vi "oscilloscope.vi"() -> ()   [LabVIEW 2023]
uses:
  <vilib>/LabVIEW Targets/FPGA/cRIO/shared/nicrio_ModuleControls/nicrio_BasicConversionTime.ctl
  <vilib>/LabVIEW Targets/FPGA/cRIO/shared/nicrio_ModuleControls/nicrio_cRIO-9775_RecordDataRates4ChansRing.ctl
  <vilib>/rvi/Emulation/niFpgaGetClockAttributes.vi
  <vilib>/rvi/Emulation/niFpgaSctlEmulationGetInTimedLoop.vi
  <vilib>/rvi/Emulation/niFpgaEmulationReportErrorSimple.vi
  <vilib>/rvi/Emulation/niFpgaProcessEmulError.vi
  <vilib>/rvi/eio/common/nirviEmuTemplateMethod_errors.vi
  <vilib>/rvi/Emulation/niFpgaCriticalErrorInLSC.vi
  <vilib>/rvi/eio/common/nirviEmuTemplatePropertySet_errors.vi
  <vilib>/eio/EIONode/EIONode.xnode
  <vilib>/eio/EIOPropertyNode/EIOPropertyNode.xnode
  <vilib>/eio/EIOMethodNode/EIOMethodNode.xnode
  <vilib>/rvi/eio/common/nirviEmuTemplatePropertyGet_errors.vi
  <vilib>/rvi/eio/common/nirviEmuTemplatePropertyGet_noerrors.vi
  <vilib>/rvi/eio/common/nirviEmuTemplatePropertySet_noerrors.vi
panel:
  in  "Reading channel":T1={"Chan 0"=TRUE, "Chan 1"=TRUE, "Chan 2"=TRUE, "Chan 3"=TRUE}
  in  "Record Samples":u32=1000000
  in  "Record Data Rate":T2=1 items=["20.000 MS/s (NI 9775)"=1, "10.00 MS/s (NI 9775)"=2, "6.667 MS/s (NI 9775)"=3, "5.000 MS/s (NI 9775)"=4, "2.500 MS/s (NI 9775)"=8, "1.667 MS/s (NI 9775)"=12, "1.250 MS/s (NI 9775)"=16, "1.000 MS/s (NI 9775)"=20, "833.333 KS/s (NI 9775)"=24, "714.286 KS/s (NI 9775)"=28, "625.000 KS/s (NI 9775)"=32, "555.556 KS/s (NI 9775)"=36, "500.000 KS/s (NI 9775)"=40, "454.545 KS/s (NI 9775)"=44, "416.667 KS/s (NI 9775)"=48, "384.615 KS/s (NI 9775)"=52, "357.143 KS/s (NI 9775)"=56, "333.333 KS/s (NI 9775)"=60, "312.500 KS/s (NI 9775)"=64, "294.118 KS/s (NI 9775)"=68, "277.778 KS/s (NI 9775)"=72, "263.158 KS/s (NI 9775)"=76, "250.000 KS/s (NI 9775)"=80, "238.095 KS/s (NI 9775)"=84, "227.273 KS/s (NI 9775)"=88, "217.391 KS/s (NI 9775)"=92, "208.333 KS/s (NI 9775)"=96, "200.000 KS/s (NI 9775)"=100, "192.308 KS/s (NI 9775)"=104, "185.185 KS/s (NI 9775)"=108, "178.571 KS/s (NI 9775)"=112, "172.414 KS/s (NI 9775)"=116, "166.667 KS/s (NI 9775)"=120, "161.290 KS/s (NI 9775)"=124, "156.250 KS/s (NI 9775)"=128, "151.515 KS/s (NI 9775)"=132, "147.059 KS/s (NI 9775)"=136, "142.857 KS/s (NI 9775)"=140, "138.889 KS/s (NI 9775)"=144, "135.135 KS/s (NI 9775)"=148, "131.579 KS/s (NI 9775)"=152, "128.205 KS/s (NI 9775)"=156, "125.000 KS/s (NI 9775)"=160, "121.951 KS/s (NI 9775)"=164, "119.048 KS/s (NI 9775)"=168, "116.279 KS/s (NI 9775)"=172, "113.636 KS/s (NI 9775)"=176, "111.111 KS/s (NI 9775)"=180, "108.696 KS/s (NI 9775)"=184, "106.383 KS/s (NI 9775)"=188, "104.167 KS/s (NI 9775)"=192, "102.041 KS/s (NI 9775)"=196, "100.000 KS/s (NI 9775)"=200, "50.000 KS/s (NI 9775)"=400, "33.333 KS/s (NI 9775)"=600, "25.000 KS/s (NI 9775)"=800, "20.000 KS/s (NI 9775)"=1000, "16.667 KS/s (NI 9775)"=1200, "14.286 KS/s (NI 9775)"=1400, "12.500 KS/s (NI 9775)"=1600, "11.111 KS/s (NI 9775)"=1800, "10.000 KS/s (NI 9775)"=2000, "9.091 KS/s (NI 9775)"=2200, "8.333 KS/s (NI 9775)"=2400, "7.692 KS/s (NI 9775)"=2600, "7.143 KS/s (NI 9775)"=2800, "6.667 KS/s (NI 9775)"=3000, "6.250 KS/s (NI 9775)"=3200, "5.882 KS/s (NI 9775)"=3400, "5.556 KS/s (NI 9775)"=3600, "5.000 KS/s (NI 9775)"=4000, "4.762 KS/s (NI 9775)"=4200, "4.545 KS/s (NI 9775)"=4400, "4.348 KS/s (NI 9775)"=4600, "4.167 KS/s (NI 9775)"=4800, "4.000 KS/s (NI 9775)"=5000, "3.846 KS/s (NI 9775)"=5200, "3.571 KS/s (NI 9775)"=5600, "3.333 KS/s (NI 9775)"=6000, "3.125 KS/s (NI 9775)"=6400, "2.941 KS/s (NI 9775)"=6800, "2.778 KS/s (NI 9775)"=7200, "2.632 KS/s (NI 9775)"=7600, "2.500 KS/s (NI 9775)"=8000, "2.381 KS/s (NI 9775)"=8400, "2.273 KS/s (NI 9775)"=8800, "2.174 KS/s (NI 9775)"=9200, "2.083 KS/s (NI 9775)"=9600, "2.000 KS/s (NI 9775)"=10000, "1.923 KS/s (NI 9775)"=10400, "1.852 KS/s (NI 9775)"=10800, "1.786 KS/s (NI 9775)"=11200, "1.724 KS/s (NI 9775)"=11600, "1.667 KS/s (NI 9775)"=12000, "1.613 KS/s (NI 9775)"=12400, "1.563 KS/s (NI 9775)"=12800, "1.515 KS/s (NI 9775)"=13200, "1.471 KS/s (NI 9775)"=13600, "1.429 KS/s (NI 9775)"=14000, "1.389 KS/s (NI 9775)"=14400, "1.351 KS/s (NI 9775)"=14800, "1.316 KS/s (NI 9775)"=15200, "1.282 KS/s (NI 9775)"=15600, "1.250 KS/s (NI 9775)"=16000, "1.220 KS/s (NI 9775)"=16400, "1.190 KS/s (NI 9775)"=16800, "1.163 KS/s (NI 9775)"=17200, "1.136 KS/s (NI 9775)"=17600, "1.111 KS/s (NI 9775)"=18000, "1.087 KS/s (NI 9775)"=18400, "1.064 KS/s (NI 9775)"=18800, "1.042 KS/s (NI 9775)"=19200, "1.020 KS/s (NI 9775)"=19600, "1.000 KS/s (NI 9775)"=20000, "0.980 KS/s (NI 9775)"=20400, "0.962 KS/s (NI 9775)"=20800, "0.943 KS/s (NI 9775)"=21200, "0.926 KS/s (NI 9775)"=21600, "0.909 KS/s (NI 9775)"=22000, "0.893 KS/s (NI 9775)"=22400, "0.877 KS/s (NI 9775)"=22800, "0.862 KS/s (NI 9775)"=23200, "0.847 KS/s (NI 9775)"=23600, "0.833 KS/s (NI 9775)"=24000, "0.820 KS/s (NI 9775)"=24400, "0.806 KS/s (NI 9775)"=24800, "0.794 KS/s (NI 9775)"=25200, "0.781 KS/s (NI 9775)"=25600, "0.694 KS/s (NI 9775)"=28800, "0.625 KS/s (NI 9775)"=32000, "0.568 KS/s (NI 9775)"=35200, "0.521 KS/s (NI 9775)"=38400, "0.446 KS/s (NI 9775)"=44800, "0.391 KS/s (NI 9775)"=51200, "0.347 KS/s (NI 9775)"=57600, "0.313 KS/s (NI 9775)"=64000]
  out "Stop":bool
  out "error out":errorcluster
  in  "Enable Low Pass Filter":T3={"Enable Low Pass Filter CH1"=TRUE, "Enable Low Pass Filter CH2"=TRUE, "Enable Low Pass Filter CH3"=TRUE, "Enable Low Pass Filter CH0"=TRUE}
  in  "Timing Mode":T4
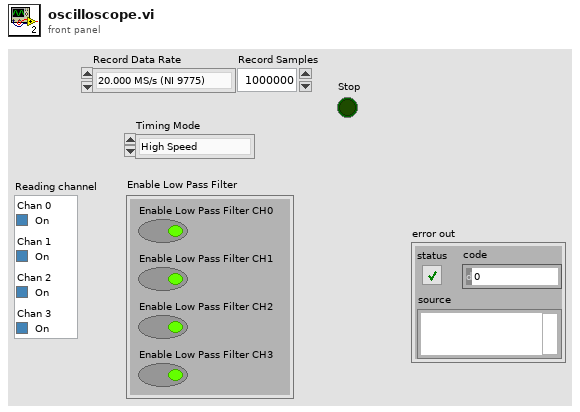
[diagram p1: front panel]
types:
  T1 = cluster{"Chan 0":bool, "Chan 1":bool, "Chan 2":bool, "Chan 3":bool}
  T2 = typedef "nicrio_cRIO-9775_RecordDataRates4ChansRing.ctl" = u16
  T3 = cluster{"Enable Low Pass Filter CH1":bool, "Enable Low Pass Filter CH2":bool, "Enable Low Pass Filter CH3":bool, "Enable Low Pass Filter CH0":bool}
  T4 = typedef "nicrio_BasicConversionTime.ctl" = enum8{"High Speed", "High Resolution"}
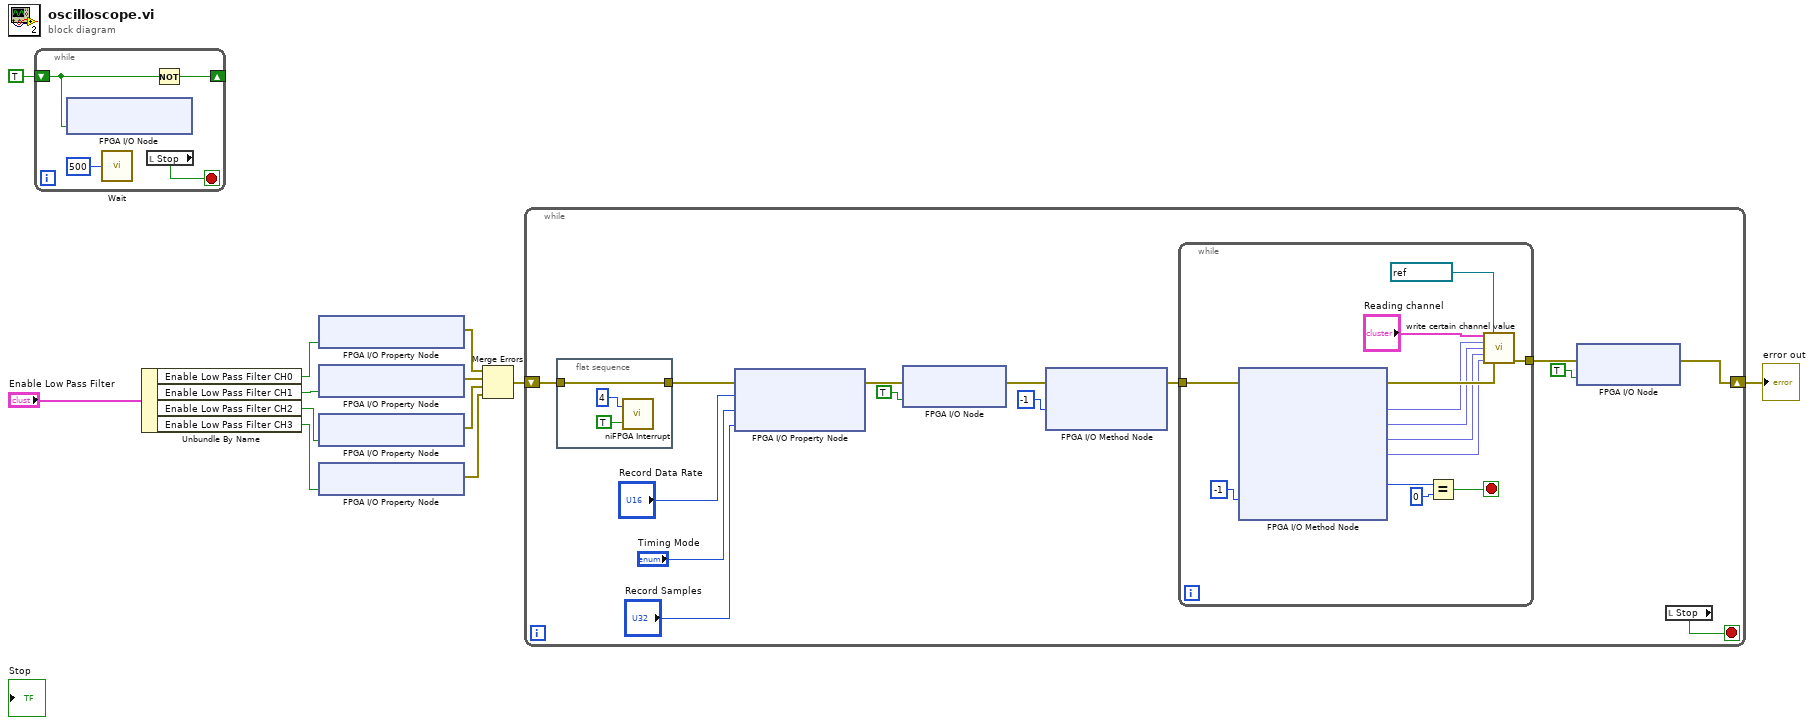
[diagram p0: block diagram]
diagram:
  n1 = while {
    shift-right: [w13] -> _
    shift-left: TRUE ("USER FPGA LED") -> [w14]
    stop <- w16 stop-if-true
    n2 = xnode "FPGA I/O Node"("USER FPGA LED"=w14) -> ()  [unwired: 1 in, 1 out]
    n3 = call "Wait"("Count(mSec)"=u32 500) -> ()  [unwired: 1 out]
    n4 = local read "Stop"() -> (w16:bool)
    n5 = Not(x=w14) -> (.not. x?=w13:bool)
  }
  n6 = Unbundle By Name("Enable Low Pass Filter") -> ("Enable Low Pass Filter CH0"=w7:bool, "Enable Low Pass Filter CH1"=w6:bool, "Enable Low Pass Filter CH2"=w5:bool, "Enable Low Pass Filter CH3"=w4:bool)
  n7 = xnode "FPGA I/O Property Node"("Enable Analog Filter"=w7) -> ("error out"=w12:errorcluster)  [unwired: 2 in, 1 out]
  n8 = xnode "FPGA I/O Property Node"("Enable Analog Filter"=w6) -> ("error out"=w11:errorcluster)  [unwired: 2 in, 1 out]
  n9 = xnode "FPGA I/O Property Node"("Enable Analog Filter"=w5) -> ("error out"=w10:errorcluster)  [unwired: 2 in, 1 out]
  n10 = xnode "FPGA I/O Property Node"("Enable Analog Filter"=w4) -> ("error out"=w9:errorcluster)  [unwired: 2 in, 1 out]
  n11 = Merge Errors(w12, w11, w10, w9) -> (w2:errorcluster)
  n12 = while {
    shift-right: [w18] -> w1
    shift-left: w2 -> [w22]
    stop <- w17 stop-if-true
    n13 = flat-sequence {
      tunnel: w22 -> [w31]
      tunnel: [w31] -> w21
      frame #0 {
        n14 = call <vilib>:"niFPGA Interrupt.vi"("Wait Until Cleared (F)"=TRUE, "IRQ Number (0)"=u8 4) -> ()  [unwired: 1 in]
      }
    }
    n15 = xnode "FPGA I/O Property Node"("error in"=w21, "Record Data Rate"="Record Data Rate", "Timing Mode"="Timing Mode", "Record Samples"="Record Samples") -> ("error out"=w27:errorcluster)  [unwired: 1 in, 1 out]
    n16 = xnode "FPGA I/O Node"("error in"=w27, "Mod1/Start"=TRUE) -> ("error out"=w20:errorcluster)  [unwired: 1 in, 1 out]
    n17 = xnode "FPGA I/O Method Node"("error in"=w20, "Timeout (Ticks)"=-1) -> ("error out"=w23:errorcluster)  [unwired: 1 in, 2 out]
    n18 = while {
      tunnel: w23 -> [w42]
      tunnel: [w34] -> w19
      stop <- w43 stop-if-true
      n19 = xnode "FPGA I/O Method Node"("error in"=w42, "Timeout (Ticks)"=-1) -> ("error out"=w41:errorcluster, "AI0"=w38:fxp<+/-,17,5>, "AI1"=w37:fxp<+/-,17,5>, "AI2"=w36:fxp<+/-,17,5>, "AI3"=w35:fxp<+/-,17,5>, "Elements Remaining"=w45:u32)  [unwired: 1 in, 3 out]
      n20 = Equal?(x=w45, y=u32 0) -> (x = y?=w43:bool)
      n21 = call "write certain channel value.vi"("Reading channel"="Reading channel", "FIFO In"=refnum<k21> "V FIFO", "Chan 0 value"=w38, "Chan 1 value"=w37, "Chan 2 value"=w36, "Chan 3 value"=w35, "error in (no error)"=w41) -> ("error out"=w34:errorcluster)  [unwired: 8 in]
    }
    n22 = xnode "FPGA I/O Node"("error in"=w19, "Mod1/Stop"=TRUE) -> ("error out"=w18:errorcluster)  [unwired: 1 in, 1 out]
    n23 = local read "Stop"() -> (w17:bool)
  }
  "error out" <- w1
